vi "Centauro LED Blinking Decider.vi"(8 "Error In":errorcluster, 10 "Blinking LED Status":T2, 11 "Normal LED Status":T2) -> (0 "Error Out":errorcluster, 3 "Final LED Status":T2)   [LabVIEW 2016]
uses:
  Centauro Washer/Product Testcode/Centauro/Valew Common/type defs/LED Status OOB.ctl
panel:
  in  "LED Status Cluster":T2
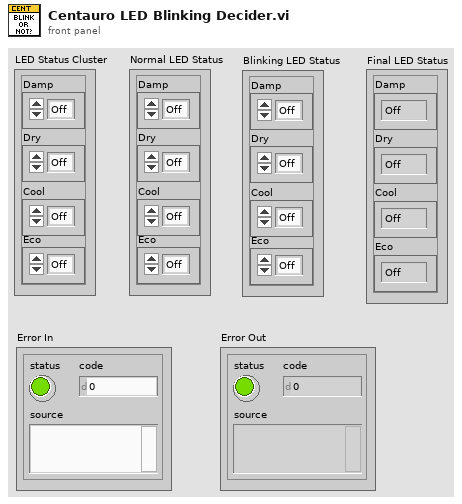
[diagram p1: front panel]
types:
  T1 = typedef "LED Status OOB.ctl" = enum32{"Off", "On", "Blink"}
  T2 = cluster{"Damp":T1, "Dry":T1, "Cool":T1, "Eco":T1}
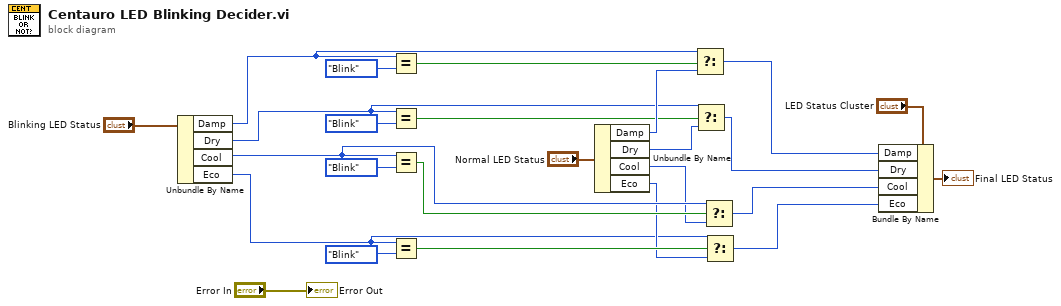
[diagram p0: block diagram]
diagram:
  n1 = Unbundle By Name("Blinking LED Status") -> ("Damp"=w18:T1, "Dry"=w14:T1, "Cool"=w12:T1, "Eco"=w8:T1)
  n2 = Equal?(x=w18, y=LED_Status_OOB."Blink" ("Damp")) -> (x = y?=w19:bool)
  n3 = Equal?(x=w14, y=LED_Status_OOB."Blink" ("Damp")) -> (x = y?=w16:bool)
  n4 = Equal?(x=w12, y=LED_Status_OOB."Blink" ("Damp")) -> (x = y?=w13:bool)
  n5 = Equal?(x=w8, y=LED_Status_OOB."Blink" ("Damp")) -> (x = y?=w10:bool)
  n6 = Unbundle By Name("Normal LED Status") -> ("Damp"=w17:T1, "Dry"=w15:T1, "Cool"=w11:T1, "Eco"=w9:T1)
  n7 = Select(t=w18, s=w19, f=w17) -> (s? t:f=w6:T1)
  n8 = Select(t=w14, s=w16, f=w15) -> (s? t:f=w5:T1)
  n9 = Select(t=w12, s=w13, f=w11) -> (s? t:f=w4:T1)
  n10 = Select(t=w8, s=w10, f=w9) -> (s? t:f=w3:T1)
  n11 = Bundle By Name(cluster="LED Status Cluster", "Damp"=w6, "Dry"=w5, "Cool"=w4, "Eco"=w3) -> (→"Final LED Status":T2)
  "Error Out" <- "Error In"
